vi "Actor Core.vi"(8 "error in":errorcluster, 11 "RandomDataChart in":refnum<class "NumericInputs.lvclass">) -> (0 "error out":errorcluster, 3 "Actor out":refnum<class "Actor.lvclass">)   [LabVIEW 2015, in "TestActors.lvlib" / "NumericInputs.lvclass"]
doc: "(<B>Filename</B>: Actor Framework.lvlib:Actor.lvclass:Actor Core.vi)\n\nReceives messages to the actor, reacts to them, and initiates any error handling that may shut the actor down.\n\nDescendant classes may override this VI to append parallel tasks for the actor to complete while it handles messages. Overrides use the Call Parent Method node."
uses:
  NumericInputs.lvclass
  <vilib>/ActorFramework/Actor/Actor.lvclass
  <vilib>/ActorFramework/Actor/Actor.lvclass/Actor.ctl
  <vilib>/ActorFramework/Message Enqueuer/Message Enqueuer.lvclass/Message Enqueuer.ctl
  <vilib>/ActorFramework/Message Enqueuer/Init from Existing Queue.vi
  IViewable/IViewable/IViewable.lvclass
  <vilib>/ActorFramework/Message Enqueuer/Message Enqueuer.lvclass
  IViewable/IViewable Messages/Broadcast DBL Msg/Broadcast DBL Msg.lvclass
panel:
  in  "Setpoint":dbl
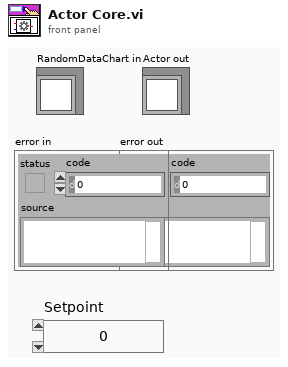
[diagram p1: front panel]
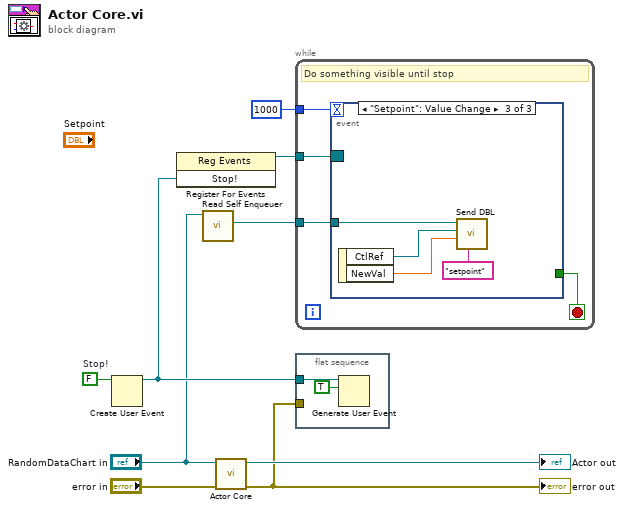
[diagram p0: block diagram]
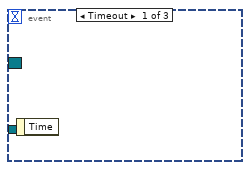
[diagram p2: hidden frame]
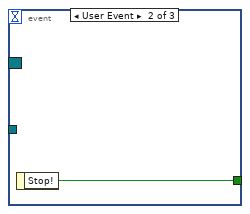
[diagram p3: hidden frame]
diagram:
  w7 = FALSE  # Stop!
  n1 = Create User Event(user event datatype=w7) -> (user event=w4:refnum<user-event>)  [unwired: 1 in, 1 out]
  n2 = register-events(w4) -> (reference out=w5:refnum<event-registration>)  [unwired: 2 in, 1 out]
  n3 = call <vilib>:"Read Self Enqueuer.vi"("Actor"="RandomDataChart in") -> ("Self Enqueuer"=w1:refnum<class "Message Enqueuer.lvclass">)  [unwired: 10 in]
  n4 = call-parent "Actor Core.vi"("error in"="error in", "IViewable In"="RandomDataChart in") -> ("error out"=w6:errorcluster, "Actor out"=→"Actor out":refnum<class "Actor.lvclass">)  [unwired: 8 in]
  "error out" <- w6
  n5 = while {
    tunnel: w5 -> [w13]
    tunnel: 1000 -> [w12]
    tunnel: w1 -> [w10]
    stop <- w11 stop-if-true
    # "Do something visible until stop"
    n6 = event shown="[2] \"Setpoint\": Value Change" {
      selector: w13 -> [_ _ _]
      dyn-events: _ -> [_ _ _]
      timeout: w12 -> [_ _ _]
      tunnel: [_ w14 _] -> w11
      tunnel: w10 -> [_ _ w18]
      event Timeout {
        n7 = event-data() -> ()  [unwired: 1 in, 1 out]
      }
      event User Event {
        n8 = event-data() -> ("Stop!"=w14:bool)  [unwired: 1 in]
      }
      event "Setpoint": Value Change {
        n9 = event-data() -> ("CtlRef"=w16:refnum<vi>, "NewVal"=w17:dbl)  [unwired: 1 in]
        n10 = call "Send DBL.vi"("Name (Use Control Label)"="setpoint" ("Name"), "Value"=w17, "DigNum Refnum"=w16, "Message Enqueuer in"=w18) -> ()  [unwired: 7 in, 1 out]
      }
    }
  }
  n11 = flat-sequence {
    tunnel: w4 -> [w20]
    tunnel: w6 -> [_]
    frame #0 {
      n12 = Generate User Event(user event=w20, event data cluster=TRUE ("event data")) -> ()  [unwired: 2 in, 2 out]
    }
  }
